vi "List.vi"(8 "error in (no error)":errorcluster) -> (0 "error out":errorcluster, 3 "Thread Names":string[](array[string]))   [LabVIEW 2018, in "Thread.lvlib"]
uses:
  Thread.lvlib
  Cache Action.ctl
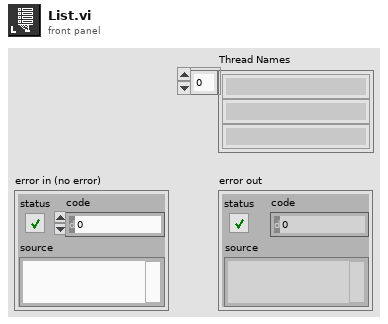
[diagram p1: front panel]
types:
  T1 = typedef "Thread.lvlib/Cache Action.ctl" = enum8{"noop", "get", "add", "remove", "remove_by_ref"}
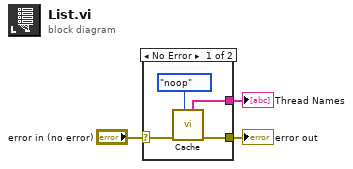
[diagram p0: block diagram]
diagram:
  n1 = case shown="No Error" "error in (no error)" {
    selector: "error in (no error)" -> [w6 w8]
    tunnel: [w5 w8] -> w2
    tunnel: [w4 _] -> w1
    frame No Error {
      n2 = call "Cache.vi"("Action"=Cache_Action."noop", "error in (no error)"=w6) -> ("error out"=w5:errorcluster, "Thread Names"=w4:string[])  [unwired: 5 in, 3 out]
    }
    frame Error {
    }
  }
  "error out" <- w2
  "Thread Names" <- w1
